vi "Remove Annotation.vi"(8 "error in (no error)":errorcluster, 10 "Name":string, 11 "FSM.Edge in":refnum<class "FSM.Edge.lvclass">) -> (0 "error out":errorcluster, 3 "FSM.Edge out":refnum<class "FSM.Edge.lvclass">)   [LabVIEW 2015, in "FSM.Edge.lvclass"]
uses:
  FSM.Edge.lvclass
  FSM.Edge.lvclass/FSM.Edge.ctl
  FSM.Annotation/FSM.Annotation.lvclass/FSM.Annotation.ctl
  FSM.Annotation/Read Items.vi
  FSM.Annotation/Write Items.vi
  FSM.Annotation/FSM.Annotation.lvclass
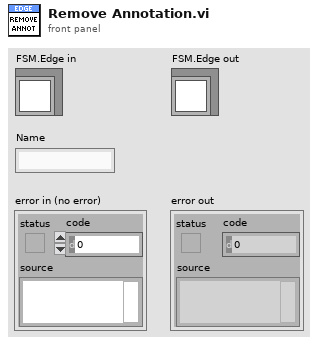
[diagram p1: front panel]
types:
  T1 = cluster{"Name":string, "Style":enum16{"Plain", "On", "Off", "On-Off"}}[]
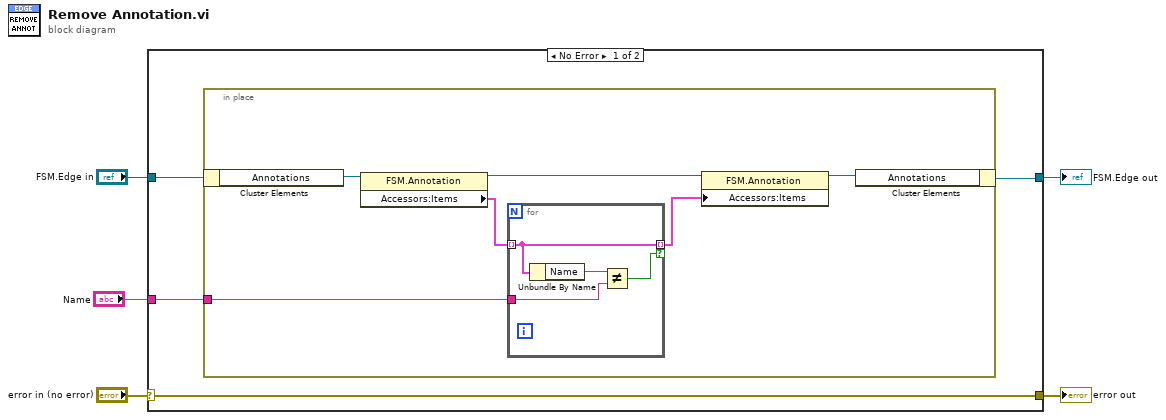
[diagram p0: block diagram]
diagram:
  n1 = case shown="No Error" "error in (no error)" {
    selector: "error in (no error)" -> [w9 w21]
    tunnel: [w9 w21] -> w4
    tunnel: [w6 w20] -> w2
    tunnel: "FSM.Edge in" -> [w8 w20]
    tunnel: "Name" -> [w7 _]
    frame No Error {
      n2 = in-place {
        in-place-border: w7 -> [w13]
        n3 = in-place-cluster #1(w8) -> ("Annotations"=w15:refnum<class "FSM.Annotation.lvclass">)
        n4 = property class="FSM.Annotation"(reference=w15) -> (reference out=w11:refnum<class "FSM.Annotation.lvclass">, "Accessors:Items"=w14:T1)  [unwired: 1 in, 1 out]
        n5 = for {
          tunnel: w14 -> [w17] mode=indexing
          tunnel: w13 -> [w18]
          tunnel: [w17] -> w10 mode=indexing if=w16
          n6 = Unbundle By Name(w17) -> ("Name"=w19:string)
          n7 = Not Equal?(x=w19, y=w18) -> (x != y?=w16:bool)
        }
        n8 = property class="FSM.Annotation"(reference=w11, "Accessors:Items"=w10) -> (reference out=w12:refnum<class "FSM.Annotation.lvclass">)  [unwired: 1 in, 1 out]
        n9 = in-place-cluster #1("Annotations"=w12) -> (w6:refnum<class "FSM.Edge.lvclass">)
      }
    }
    frame Error {
    }
  }
  "error out" <- w4
  "FSM.Edge out" <- w2
